vi "Create Shared Data DVR.vi"(8 "error in (no error)":errorcluster) -> (0 "error out":errorcluster, 3 "Shared Data DVR":T1)   [LabVIEW 2017, in "DSF System Explorer.lvlib"]
uses:
  DSF System Explorer.lvlib
  shared data ref.ctl
  shared data.ctl
  DSF Core.lvlibp/Classes/Configuration/Configuration Session.lvclass
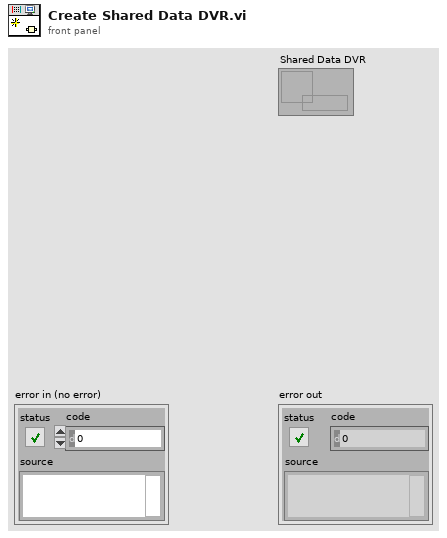
[diagram p1: front panel]
types:
  T1 = typedef "DSF System Explorer.lvlib/shared data ref.ctl" = refnum<data-value>
  T2 = typedef "DSF System Explorer.lvlib/shared data.ctl" = cluster{"Configuration Session":refnum<class "Configuration Session.lvclass">}
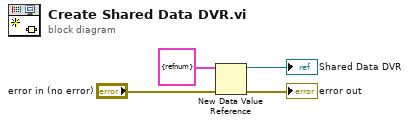
[diagram p0: block diagram]
diagram:
  n1 = New Data Value Reference(data value=T2 {"Configuration Session"=refnum} ("Shared Data"), error in="error in (no error)") -> (data value reference=→"Shared Data DVR":refnum<data-value>, error out=→"error out":errorcluster)
